vi "SimpleAdvancedSequence.vi"() -> ()   [LabVIEW 2023]
uses:
  <instrlib>/niDCPower/nidcpower.llb/niDCPower Sequence Attribute Type.ctl
  <instrlib>/niDCPower/nidcpower.llb/niDCPower Source Mode.ctl
  <instrlib>/niDCPower/nidcpower.llb/niDCPower Output Function.ctl
  <instrlib>/niDCPower/nidcpower.llb/niDCPower Create Advanced Sequence Step With Channels.vi
panel:
  out "Waveform Chart":dbl[](graph)
  in  "SequenceSettings":T1(array[cluster])=[{"Source:DC Voltage:Voltage Level"=0.0, "Source:DC Voltage:Current Limit"=0.0, "Source:DC Voltage:Current Limit Range"=0.0}, {"Source:DC Voltage:Voltage Level"=0.0, "Source:DC Voltage:Current Limit"=0.0, "Source:DC Voltage:Current Limit Range"=0.0}, {"Source:DC Voltage:Voltage Level"=2.0, "Source:DC Voltage:Current Limit"=0.0, "Source:DC Voltage:Current Limit Range"=0.0}, {"Source:DC Voltage:Voltage Level"=4.0, "Source:DC Voltage:Current Limit"=0.0, "Source:DC Voltage:Current Limit Range"=0.0}, {"Source:DC Voltage:Voltage Level"=0.0, "Source:DC Voltage:Current Limit"=0.0, "Source:DC Voltage:Current Limit Range"=0.0}]
  out "error out":errorcluster
  in  "resource name":refnum<k15>
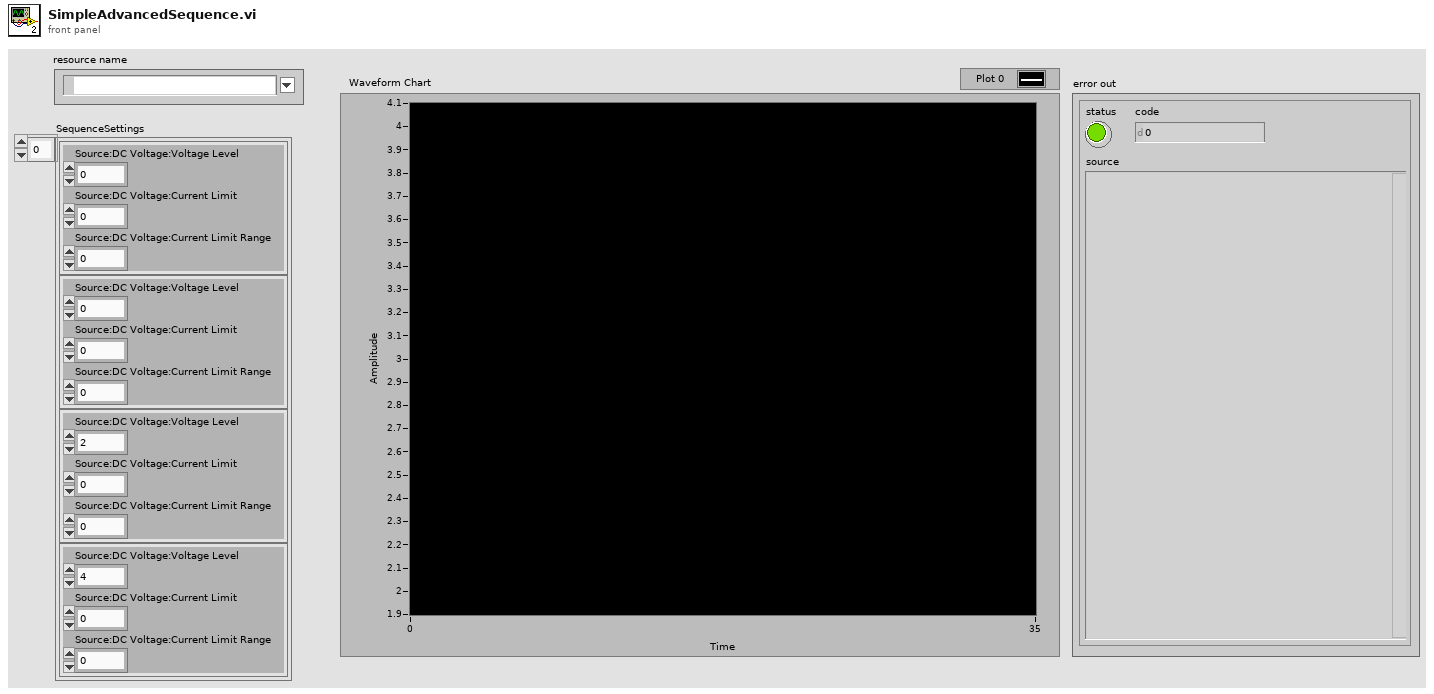
[diagram p1: front panel]
types:
  T1 = cluster{"Source:DC Voltage:Voltage Level":dbl, "Source:DC Voltage:Current Limit":dbl, "Source:DC Voltage:Current Limit Range":dbl}[]
  T2 = typedef "niDCPower Output Function.ctl" = i32
  T3 = typedef "niDCPower Source Mode.ctl" = i32
  T4 = typedef "niDCPower Sequence Attribute Type.ctl" = i32
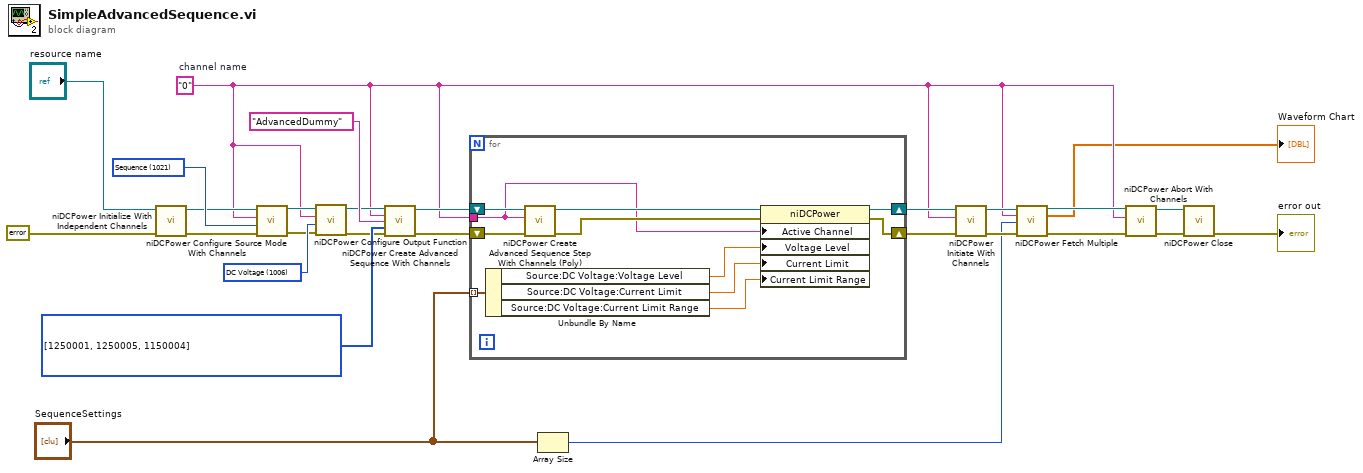
[diagram p0: block diagram]
diagram:
  w9 = T2 1006 items=["DC Voltage"=1006, "DC Current"=1007, "Pulse Voltage"=1049, "Pulse Current"=1050] ("output function")
  w12 = T3 1021 items=["Single Point"=1020, "Sequence"=1021] ("source mode")
  w14 = T4[] [1250001, 1250005, 1150004] items=["Source -> Output Function"=1150008, "Source -> Output Enabled"=1250006, "Source -> Output Resistance"=1150061, "Source -> Transient Response"=1150062, "Source -> Custom Transient Response -> Voltage Gain Bandwidth"=1150067, "Source -> Custom Transient Response -> Voltage Compensation Frequency"=1150068, "Source -> Custom Transient Response -> Voltage Pole-Zero Ratio"=1150069, "Source -> Custom Transient Response -> Current Gain Bandwidth"=1150070, "Source -> Custom Transient Response -> Current Compensation Frequency"=1150071, "Source -> Custom Transient Response -> Current Pole-Zero Ratio"=1150072, "Source -> DC Voltage -> Voltage Level"=1250001, "Source -> DC Voltage -> Voltage Level Range"=1150005, "Source -> DC Voltage -> Current Limit"=1250005, "Source -> DC Voltage -> Current Limit High"=1150187, "Source -> DC Voltage -> Current Limit Low"=1150188, "Source -> DC Voltage -> Current Limit Range"=1150004, "Source -> DC Current -> Current Level"=1150009, "Source -> DC Current -> Current Level Range"=1150011, "Source -> DC Current -> Voltage Limit"=1150010, "Source -> DC Current -> Voltage Limit High"=1150185, "Source -> DC Current -> Voltage Limit Low"=1150186, "Source -> DC Current -> Voltage Limit Range"=1150012, "Source -> DC Current -> Current Level Slew Rate -> Rising"=1150343, "Source -> DC Current -> Current Level Slew Rate -> Falling"=1150344, "Source -> Pulse Voltage -> Pulse Voltage Level"=1150080, "Source -> Pulse Voltage -> Pulse Bias Voltage Level"=1150082, "Source -> Pulse Voltage -> Pulse Voltage Level Range"=1150084, "Source -> Pulse Voltage -> Pulse Current Limit"=1150081, "Source -> Pulse Voltage -> Pulse Current Limit High"=1150193, "Source -> Pulse Voltage -> Pulse Current Limit Low"=1150194, "Source -> Pulse Voltage -> Pulse Bias Current Limit"=1150083, "Source -> Pulse Voltage -> Pulse Bias Current Limit High"=1150195, "Source -> Pulse Voltage -> Pulse Bias Current Limit Low"=1150196, "Source -> Pulse Voltage -> Pulse Current Limit Range"=1150085, "Source -> Pulse Current -> Pulse Current Level"=1150086, "Source -> Pulse Current -> Pulse Bias Current Level"=1150088, "Source -> Pulse Current -> Pulse Current Level Range"=1150090, "Source -> Pulse Current -> Pulse Voltage Limit"=1150087, "Source -> Pulse Current -> Pulse Voltage Limit High"=1150189, "Source -> Pulse Current -> Pulse Voltage Limit Low"=1150190, "Source -> Pulse Current -> Pulse Bias Voltage Limit"=1150089, "Source -> Pulse Current -> Pulse Bias Voltage Limit High"=1150191, "Source -> Pulse Current -> Pulse Bias Voltage Limit Low"=1150192, "Source -> Pulse Current -> Pulse Voltage Limit Range"=1150091, "Source -> Advanced -> Source Delay"=1150051, "Source -> Advanced -> Pulse Bias Delay"=1150092, "Source -> Advanced -> Pulse On Time"=1150093, "Source -> Advanced -> Pulse Off Time"=1150094, "Source -> Advanced -> OVP Enabled"=1250002, "Source -> Advanced -> OVP Limit"=1250003, "Source -> Advanced -> Compliance Limit Symmetry"=1150184, "Source -> Advanced -> Sequence Step Delta Time"=1150198, "Source -> Advanced -> Conduction Voltage -> Mode"=1150350, "Source -> Advanced -> Conduction Voltage -> On Threshold"=1150351, "Source -> Advanced -> Conduction Voltage -> Off Threshold"=1150352, "Measurement -> Sense"=1150013, "Measurement -> Aperture Time"=1150058, "Measurement -> Measure Record Length"=1150063, "Measurement -> Advanced -> DC Noise Rejection"=1150066, "Measurement -> Autorange"=1150244, "Measurement -> Advanced -> Autorange Behavior"=1150245, "Measurement -> Advanced -> Autorange Aperture Time Mode"=1150246, "Measurement -> Advanced -> Autorange Minimum Aperture Time"=1150247, "Measurement -> Advanced -> Autorange Minimum Aperture Time Units"=1150248, "Measurement -> Advanced -> Autorange Minimum Current Range"=1150255, "Measurement -> Advanced -> Autorange Minimum Voltage Range"=1150256, "Measurement -> Advanced -> Autorange Threshold Mode"=1150257, "Measurement -> Advanced -> Autorange Maximum Delay After Range Change"=1150322, "LCR -> Instrument Mode"=1150208, "LCR -> Source Delay Mode"=1150315, "LCR -> Measurement Time"=1150218, "LCR -> Custom Measurement Time"=1150258, "LCR -> AC Stimulus -> Function"=1150209, "LCR -> AC Stimulus -> Frequency"=1150210, "LCR -> AC Stimulus -> Voltage Amplitude"=1150211, "LCR -> AC Stimulus -> Current Amplitude"=1150212, "LCR -> AC Stimulus -> Advanced -> Voltage Range"=1150265, "LCR -> AC Stimulus -> Advanced -> Current Range"=1150267, "LCR -> AC Stimulus -> Advanced -> Source Aperture Time"=1150349, "LCR -> DC Bias -> Source"=1150213, "LCR -> DC Bias -> Voltage Level"=1150214, "LCR -> DC Bias -> Current Level"=1150215, "LCR -> DC Bias -> Advanced -> Voltage Range"=1150266, "LCR -> DC Bias -> Advanced -> Current Range"=1150274, "LCR -> DC Bias -> Advanced -> Transient Response"=1150347, "LCR -> Compensation -> Open -> Enabled"=1150220, "LCR -> Compensation -> Open -> Conductance"=1150261, "LCR -> Compensation -> Open -> Susceptance"=1150262, "LCR -> Compensation -> Short -> Enabled"=1150221, "LCR -> Compensation -> Short -> Resistance"=1150263, "LCR -> Compensation -> Short -> Reactance"=1150264, "LCR -> Compensation -> Load -> Enabled"=1150222, "LCR -> Compensation -> Load -> Measured Resistance"=1150268, "LCR -> Compensation -> Load -> Measured Reactance"=1150269, "LCR -> Compensation -> Load -> Actual Resistance"=1150270, "LCR -> Compensation -> Load -> Actual Reactance"=1150271, "LCR -> Impedance Range -> Impedance Range"=1150217, "LCR -> Impedance Range -> Impedance Autorange"=1150216, "LCR -> Impedance Range -> Advanced -> Impedance Range Source"=1150321, "LCR -> Impedance Range -> Advanced -> Load Resistance"=1150318, "LCR -> Impedance Range -> Advanced -> Load Inductance"=1150319, "LCR -> Impedance Range -> Advanced -> Load Capacitance"=1150320] ("advanced sequence properties")
  w4 = "0"  # channel name
  n1 = call <instrlib>:"niDCPower Initialize With Independent Channels.vi"("error in (no error)"=errorcluster {"status"=FALSE, "code"=0, "source"=""}, "resource name"="resource name") -> ("error out"=w10:errorcluster, "instrument handle out"=w11:refnum<k15>)  [unwired: 8 in]
  n2 = call <instrlib>:"niDCPower Configure Source Mode With Channels.vi"("error in (no error)"=w10, "source mode"=w12, "channel name"=w4, "instrument handle"=w11) -> ("error out"=w5:errorcluster, "instrument handle out"=w8:refnum<k15>)  [unwired: 6 in]
  n3 = call <instrlib>:"niDCPower Configure Output Function.vi"("error in (no error)"=w5, "output function"=w9, "channel name"=w4, "instrument handle"=w8) -> ("error out"=w6:errorcluster, "instrument handle out"=w7:refnum<k15>)  [unwired: 6 in]
  n4 = call <instrlib>:"niDCPower Create Advanced Sequence With Channels.vi"("instrument handle"=w7, "channel name"=w4, "sequence name"="AdvancedDummy", "advanced sequence properties"=w14, "error in (no error)"=w6) -> ("instrument handle out"=w25:refnum<k15>, "error out"=w24:errorcluster)  [unwired: 9 in]
  n5 = for {
    tunnel: w4 -> [w32]
    shift-right: [w33] -> w23
    shift-left: w25 -> [w38]
    shift-right: [w34] -> w22
    shift-left: w24 -> [w37]
    tunnel: "SequenceSettings" -> [w31] mode=indexing
    n6 = Unbundle By Name(w31) -> ("Source:DC Voltage:Voltage Level"=w30:dbl, "Source:DC Voltage:Current Limit"=w29:dbl, "Source:DC Voltage:Current Limit Range"=w28:dbl)
    n7 = call-poly <instrlib>:"niDCPower Create Advanced Sequence Step With Channels (Poly).vi"("error in (no error)"=w37, "channel name"=w32, "instrument handle"=w38) -> ("error out"=w36:errorcluster, "instrument handle out"=w35:refnum<k15>)  [unwired: 7 in]
    n8 = property class="niDCPower"(reference=w35, error in=w36, "Active Channel"=w32, "Voltage Level"=w30, "Current Limit"=w29, "Current Limit Range"=w28) -> (reference out=w33:refnum<k15>, error out=w34:errorcluster)
  }
  n9 = Array Size(array="SequenceSettings") -> (size(s)=w1:i32)
  n10 = call <instrlib>:"niDCPower Initiate With Channels.vi"("error in (no error)"=w22, "channel name"=w4, "instrument handle"=w23) -> ("error out"=w20:errorcluster, "instrument handle out"=w21:refnum<k15>)  [unwired: 7 in]
  n11 = call <instrlib>:"niDCPower Fetch Multiple.vi"("instrument handle"=w21, "channel name"=w4, "count (1)"=w1, "error in (no error)"=w20) -> ("instrument handle out"=w27:refnum<k15>, "voltage measurements"=→"Waveform Chart":dbl[], "error out"=w26:errorcluster)  [unwired: 6 in, 3 out]
  n12 = call <instrlib>:"niDCPower Abort With Channels.vi"("error in (no error)"=w26, "channel name"=w4, "instrument handle"=w27) -> ("error out"=w18:errorcluster, "instrument handle out"=w19:refnum<k15>)  [unwired: 7 in]
  n13 = call <instrlib>:"niDCPower Close.vi"("error in (no error)"=w18, "instrument handle"=w19) -> ("error out"=→"error out":errorcluster)  [unwired: 9 in]
